vi "tio32_AdsMux.vi"(0 "VISA resource name":refnum<visa-resource-name>, 5 "Board address":i32=4660 format="%x", 7 "MUX number":i32=1, 11 "error in (no error)":errorcluster, 12 "Input P":i32=1, 13 "Input N":i32=1) -> (4 "VISA resource name out":refnum<visa-resource-name>, 6 "return":i32=666, 15 "error out":errorcluster)   [LabVIEW 2011]
uses:
  l_pse_dll/Tio32.dll
panel:
  # "tio32_AdsMux"
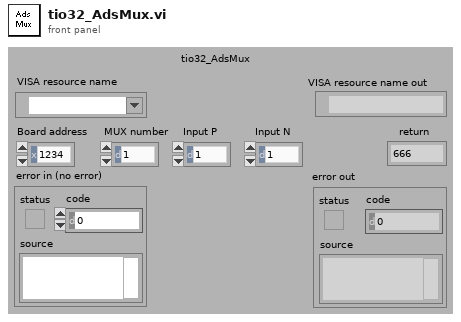
[diagram p1: front panel]
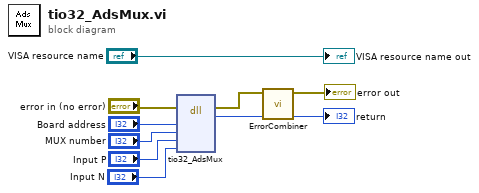
[diagram p0: block diagram]
diagram:
  n1 = dll-call lib="C:/Users/Ikaika's/Documents/DCC/Apps/INA231/INA231-SFT-rev1/INA231-Sourcecode-rev1/INA231/Shell Resources/l_pse_dll/Tio32.dll" fn="tio32_AdsMux" label="tio32_AdsMux()"(error in="error in (no error)", "adr"="Board address", "muxNo"="MUX number", "in_p"="Input P", "in_n"="Input N") -> (error out=w5:errorcluster, "Rückgabetyp"=w6:i32)  [unwired: 6 in, 1 out]
  n2 = call "ErrorCombiner.vi"("Return In"=w6, "error in (no error)"=w5) -> ("Return Out"=→"return":i32, "error out"=→"error out":errorcluster)  [unwired: 8 in]
  "VISA resource name out" <- "VISA resource name"
